vi "Update_UI.vi"(8 "error in (no error)":errorcluster, 10 "srcsettings":T1, 11 "IB_Settings_Item_File in":refnum<class "IB_Settings_Item_File.lvclass">) -> (0 "error out":errorcluster, 2 "validate permisions?":bool, 3 "IB_Settings_Item_File out":refnum<class "IB_Settings_Item_File.lvclass">)   [LabVIEW 2020, in "IB_Settings_Item_File.lvclass"]
uses:
  <vilib>/AppBuilder/IB_Classes/Settings_Item_File/IB_Settings_Item_File.lvclass
  <vilib>/AppBuilder/IB_Classes/Settings_Item_File/IB_Settings_Item_File.lvclass/IB_Settings_Item_File.ctl
  <vilib>/AppBuilder/IB_Classes/Settings_Item/IB_Settings_Item.lvclass
  e:/builds/penguin/labview/branches/2020/dev/dist/vi.lib/AppBuilder/IB_Classes/Settings_Item/IB_Settings_Item.lvclass
  e:/builds/penguin/labview/branches/2020/dev/dist/vi.lib/AppBuilder/IB_Classes/Settings_Item_File/IB_Settings_Item_File.lvclass
  <resource>/Framework/Providers/Builds/Installer/CDK_sTypeDef_FILEATTRIBUTES.ctl
  <resource>/Framework/Providers/Builds/Installer/Pages/controls/IB_UI_Page_SrcSettings_References.ctl
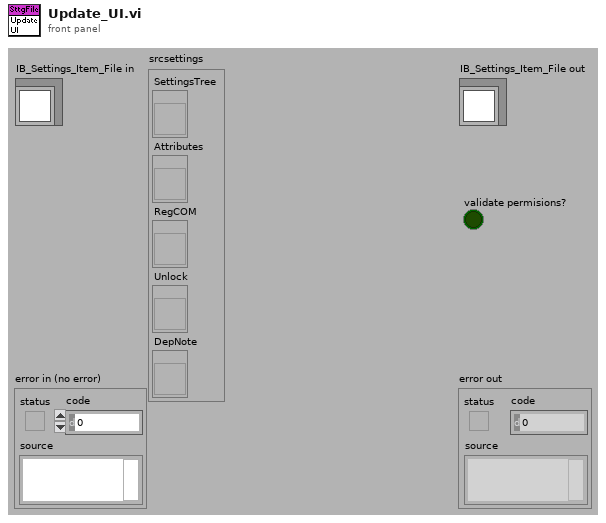
[diagram p1: front panel]
types:
  T1 = typedef "IB_UI_Page_SrcSettings_References.ctl" = cluster{"SettingsTree":refnum<vi>, "Attributes":refnum<vi>, "RegCOM":refnum<vi>, "Unlock":refnum<vi>, "DepNote":refnum<vi>}
  T2 = enum8{"Enabled", "Disabled", "Disabled and Grayed Out"}
  T3 = typedef "IB_Settings_Item.ctl" = cluster{"address":string[], "Attributes":i16, "RegCOM":bool, "unlock":bool}
  T4 = typedef "CDK_sTypeDef_FILEATTRIBUTES.ctl" = cluster{"fAttribute":bool, "fAttribute 2":bool, "fAttribute 3":bool, "fAttribute 4":bool}
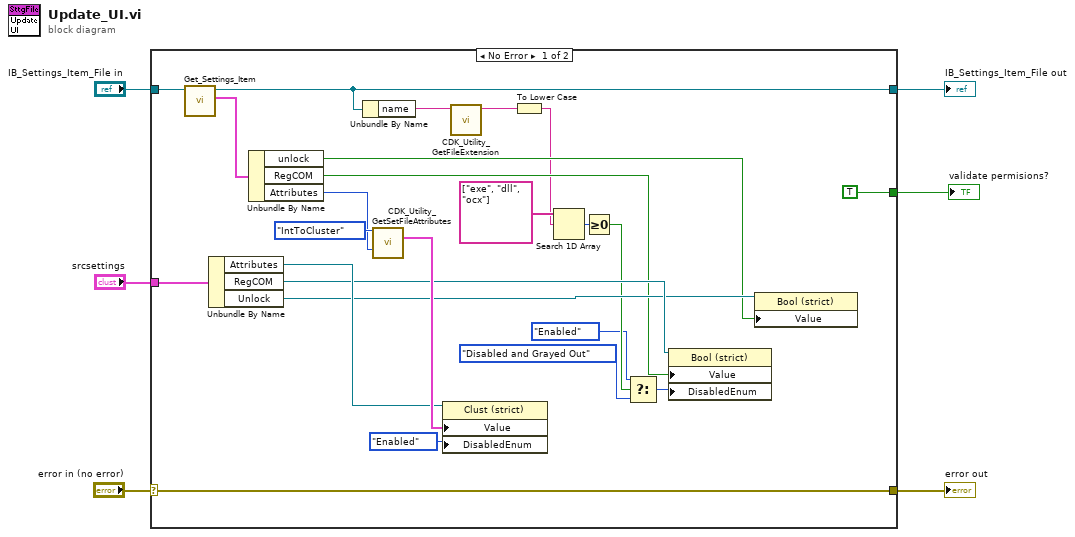
[diagram p0: block diagram]
diagram:
  n1 = case shown="No Error" "error in (no error)" {
    selector: "error in (no error)" -> [w30 w32]
    tunnel: [w30 w32] -> w5
    tunnel: "srcsettings" -> [w28 _]
    tunnel: "IB_Settings_Item_File in" -> [w16 w31]
    tunnel: [w15 w31] -> w2
    tunnel: [TRUE _] -> w1
    frame No Error {
      n2 = call <vilib>:"Get_Settings_Item.vi"("IB_Settings_Item in"=w16) -> ("data"=w29:T3, "IB_Settings_Item out"=w15:refnum<class "IB_Settings_Item_File.lvclass">)  [unwired: 1 in, 8 out]
      n3 = Unbundle By Name(w28) -> ("Attributes"=w24:refnum<vi>, "RegCOM"=w22:refnum<vi>, "Unlock"=w21:refnum<vi>)
      n4 = Unbundle By Name(w29) -> ("unlock"=w19:bool, "RegCOM"=w20:bool, "Attributes"=w26:i16)
      n5 = Unbundle By Name(w15) -> ("name"=w9:string)
      n6 = call <resource>:"CDK_Utility_GetSetFileAttributes.vi"("Action"=enum16{"ClusterToInt", "IntToCluster"}."IntToCluster", "FileAttribIn"=w26) -> ("AttribOut"=w25:T4)  [unwired: 2 in, 11 out]
      n7 = property class="Clust (strict)"(reference=w24, "Value"=w25, "DisabledEnum"=T2."Enabled" ("Disabled")) -> ()  [unwired: 1 in, 2 out]
      n8 = call <resource>:"CDK_Utility_GetFileExtension.vi"("filename"=w9) -> ("extension"=w8:string)  [unwired: 10 out]
      n9 = To Lower Case(string=w8) -> (all lower case string=w10:string)
      n10 = Search 1D Array(1D array=string[] ["exe", "dll", "ocx"], element=w10) -> (index of element=w18:i32)  [unwired: 1 out]
      n11 = Greater Or Equal To 0?(x=w18) -> (x >= 0?=w13:bool)
      n12 = Select(t=T2."Enabled" ("Disabled"), s=w13, f=T2."Disabled and Grayed Out" ("Disabled")) -> (s? t:f=w14:T2)
      n13 = property class="Bool (strict)"(reference=w22, "Value"=w20, "DisabledEnum"=w14) -> ()  [unwired: 1 in, 2 out]
      n14 = property class="Bool (strict)"(reference=w21, "Value"=w19) -> ()  [unwired: 1 in, 2 out]
    }
    frame Error {
    }
  }
  "error out" <- w5
  "IB_Settings_Item_File out" <- w2
  "validate permisions?" <- w1
